vi "EOL Digital Inputs v2.vi"(8 "Sys Error In":errorcluster, 9 "Digital Inputs Array":T1[](array[typedef]), 10 "DI Map path":path=path "C:/Labview Code/System/Digital Input Channel Configuration", 11 "Mode":enum16{"Init", "Read", "Read All", "Close"}(ring)) -> (0 "Sys Error Out":errorcluster, 2 "Single Input":bool, 3 "DI Status":bool[](array[boolean]))   [LabVIEW 2018]
uses:
  05.UserVI's/type defs/EOL Global Digital Input Control.ctl
  <vilib>/DAQmx/read.llb/DAQmx Read (Digital 1D Bool NChan 1Samp 1Line).vi
  <vilib>/DAQmx/miscellaneous.llb/DAQmx Fill In Error Info.vi
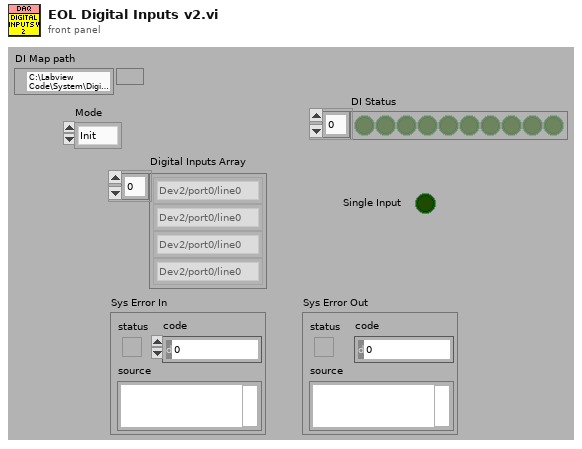
[diagram p1: front panel]
types:
  T1 = typedef "EOL Global Digital Input Control.ctl" = enum16{"Dev2/port0/line0", "Dev2/port0/line1", "Dev2/port0/line2", "Dev2/port0/line3", "Dev2/port0/line4", "Dev2/port0/line5", "Dev2/port0/line6", "Dev2/port0/line7", "Dev2/port1/line0", "Dev2/port1/line1", "Dev2/port1/line2", "Dev2/port1/line3", "Dev2/port1/line4", "Dev2/port1/line5", "Dev2/port1/line6", "Dev2/port1/line7", "Dev2/port2/line0", "Dev2/port2/line1", "Dev2/port2/line2", "Dev2/port2/line3", "Dev2/port2/line4", "Dev2/port2/line5", "Dev2/port2/line6", "Dev2/port2/line7", "Prerun Start Test", "Prerun Abort Test", "Audit Start Test", "Audit Abort Test", "Dev2/port3/line4", "Dev2/port3/line5", "Breakin Start Test", "Breakin Abort Test", "Not Implemented"}
  T2 = cluster{"DI Task":refnum<k21>, "DI Status":bool[], "Error":errorcluster}
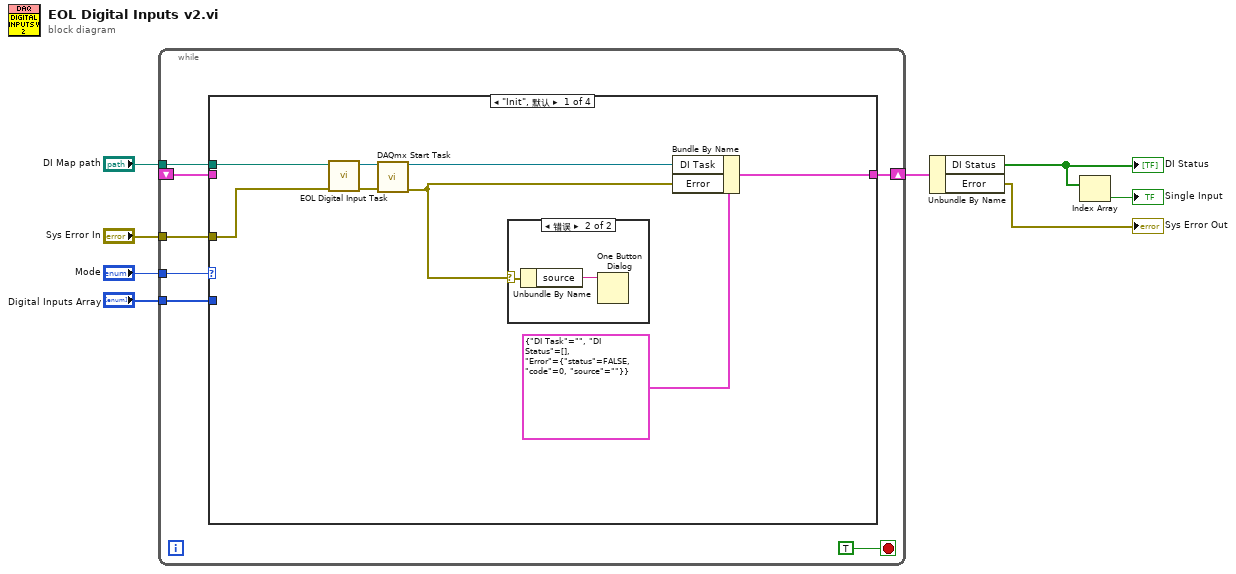
[diagram p0: block diagram]
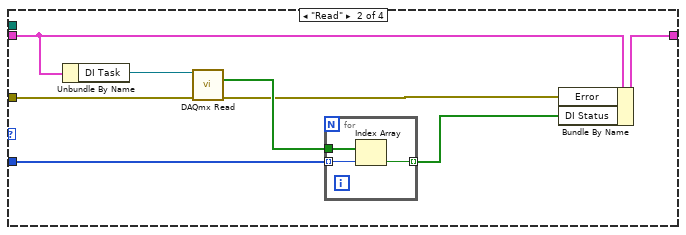
[diagram p3: hidden frame]
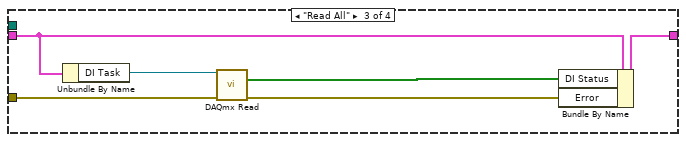
[diagram p4: hidden frame]
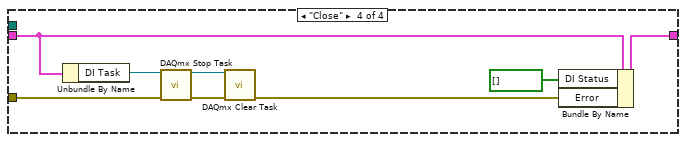
[diagram p5: hidden frame]
diagram:
  n1 = while {
    tunnel: "Mode" -> [w14]
    tunnel: "Digital Inputs Array" -> [w13]
    shift-right: [w12] -> w6
    shift-left: _ -> [w11]
    tunnel: "Sys Error In" -> [w10]
    tunnel: "DI Map path" -> [w9]
    stop <- TRUE stop-if-true
    n2 = case shown="\"Init\", 默认" w14 {
      tunnel: w13 -> [_ w32 _ _]
      tunnel: [w22 w29 w40 w48] -> w12
      tunnel: w11 -> [_ w30 w41 w49]
      tunnel: w10 -> [w18 w26 w37 w43]
      tunnel: w9 -> [w16 _ _ _]
      frame "Init", Default {
        n3 = call "EOL Digital Input Task.vi"("error in"=w18, "path"=w16) -> ("error out"=w17:errorcluster, "DI Task"=w19:refnum<k21>)  [unwired: 8 in]
        n4 = call <vilib>:"DAQmx Start Task.vi"("task/channels in"=w19, "error in"=w17) -> ("task out"=w21:refnum<k21>, "error out"=w20:errorcluster)  [unwired: 12 in]
        n5 = case shown="错误" w20 {
          selector: w20 -> [_ w25]
          frame No Error {
          }
          frame Error {
            n6 = Unbundle By Name(w25) -> ("source"=w24:string)
            n7 = One Button Dialog(message=w24) -> ()  [unwired: 1 in, 1 out]
          }
        }
        n8 = Bundle By Name(cluster=T2 {"DI Task"="", "DI Status"=[], "Error"={"status"=FALSE, "code"=0, "source"=""}}, "DI Task"=w21, "Error"=w20) -> (w22:T2)
      }
      frame "Read" {
        n9 = Unbundle By Name(w30) -> ("DI Task"=w33:refnum<k21>)
        n10 = call-poly <vilib>:"DAQmx Read.vi"("task/channels in"=w33, "error in"=w26) -> ("data"=w31:bool[], "error out"=w28:errorcluster)  [unwired: 11 in, 1 out]
        n11 = for {
          tunnel: w32 -> [w36] mode=indexing
          tunnel: [w35] -> w27 mode=indexing
          tunnel: w31 -> [w34]
          n12 = Index Array(array=w34, index=w36) -> (element=w35:bool)
        }
        n13 = Bundle By Name(cluster=w30, "Error"=w28, "DI Status"=w27) -> (w29:T2)
      }
      frame "Read All" {
        n14 = Unbundle By Name(w41) -> ("DI Task"=w42:refnum<k21>)
        n15 = call-poly <vilib>:"DAQmx Read.vi"("task/channels in"=w42, "error in"=w37) -> ("data"=w39:bool[], "error out"=w38:errorcluster)  [unwired: 11 in, 1 out]
        n16 = Bundle By Name(cluster=w41, "DI Status"=w39, "Error"=w38) -> (w40:T2)
      }
      frame "Close" {
        n17 = Unbundle By Name(w49) -> ("DI Task"=w50:refnum<k21>)
        n18 = call <vilib>:"DAQmx Stop Task.vi"("task/channels in"=w50, "error in"=w43) -> ("task out"=w46:refnum<k21>, "error out"=w45:errorcluster)  [unwired: 12 in]
        n19 = call <vilib>:"DAQmx Clear Task.vi"("task in"=w46, "error in"=w45) -> ("error out"=w44:errorcluster)  [unwired: 13 in]
        n20 = Bundle By Name(cluster=w49, "DI Status"=bool[] [], "Error"=w44) -> (w48:T2)
      }
    }
  }
  n21 = Unbundle By Name(w6) -> ("DI Status"=w5:bool[], "Error"=→"Sys Error Out":errorcluster)
  "DI Status" <- w5
  n22 = Index Array(array=w5) -> (element=→"Single Input":bool)  [unwired: 1 in]
